vi "Prog_Revision_Date.vi"(5 "Input string":string) -> (0 "Revision time (s)":u32, 2 "svnBaseRevision":u32, 3 "Prog's last revision date":string)   [LabVIEW 2011]
uses:
  <vilib>/Utility/miscctls.llb/LVDateTimeRec.ctl
panel:
  out "source":string
  out "Prog's last revision time":string
  out "RevisionData":string
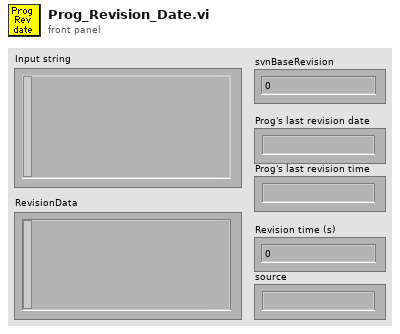
[diagram p1: front panel]
types:
  T1 = typedef "LVDateTimeRec.ctl" = cluster{"fractional second":dbl, "second":i32, "minute":i32, "hour":i32, "day of month":i32, "month":i32, "year":i32, "day of week":i32, "day of year":i32, "DST":i32}
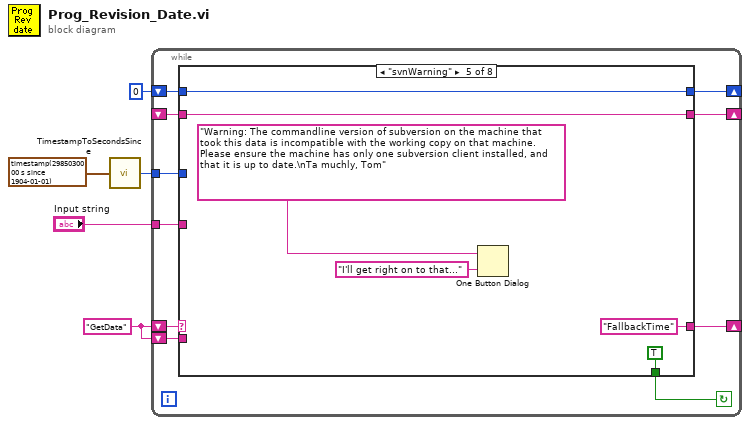
[diagram p0: block diagram]
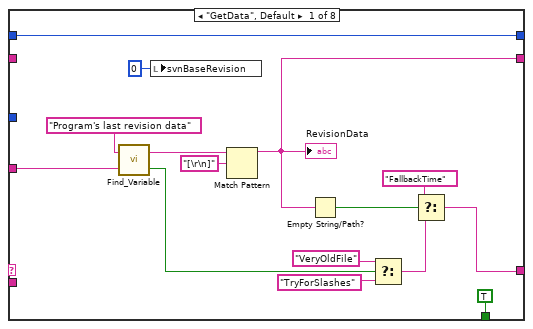
[diagram p2: hidden frame]
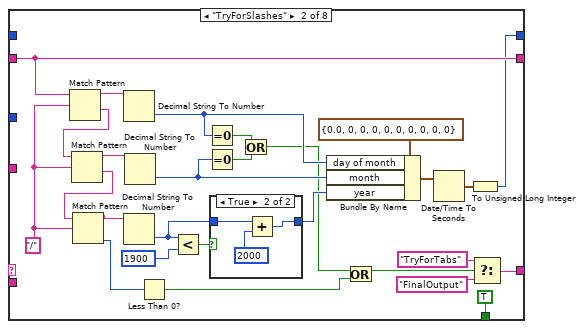
[diagram p3: hidden frame]
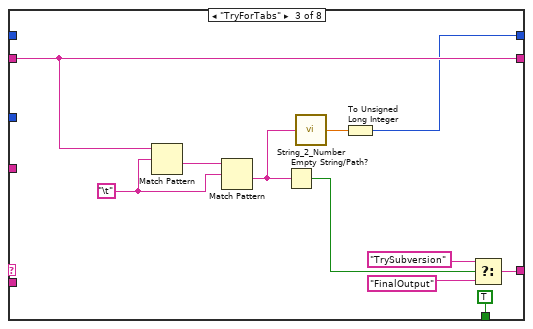
[diagram p5: hidden frame]
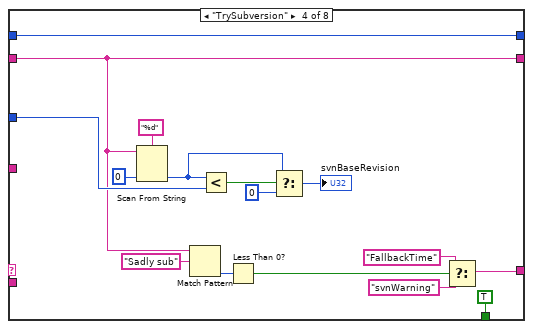
[diagram p6: hidden frame]
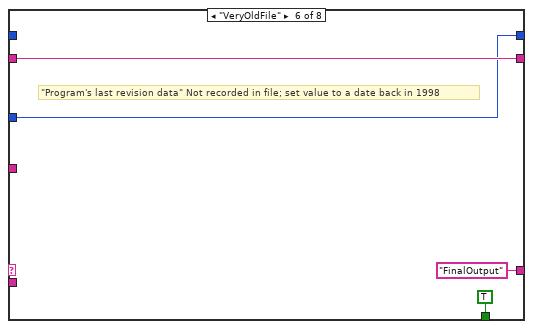
[diagram p7: hidden frame]
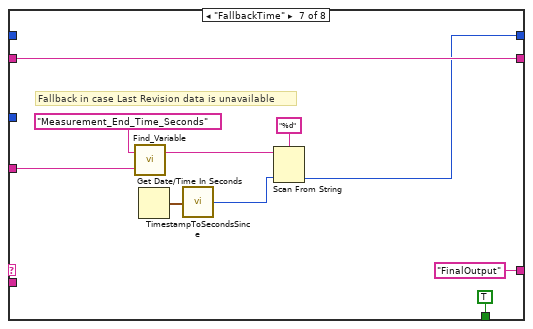
[diagram p8: hidden frame]
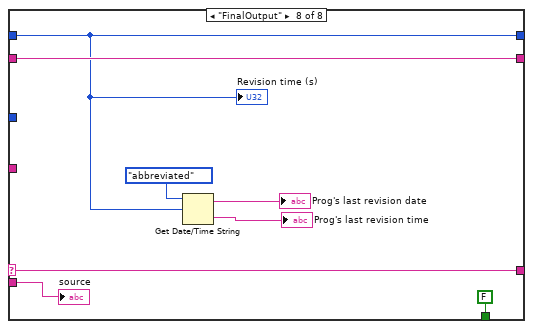
[diagram p9: hidden frame]
diagram:
  w1 = "GetData"
  n1 = call "TimestampToSecondsSince.vi"("Time Stamp Control"=timestamp(2985030000 s since 1904-01-01)) -> ("unsigned 32bit integer"=w2:u32)
  n2 = while {
    tunnel: "Input string" -> [w15]
    shift-right: [w13] -> _
    shift-left: w1 -> [w14]
    shift-right: [w12] -> _
    shift-left: u32 0 -> [w11]
    shift-right: [w9] -> _
    shift-left: _ -> [w8]
    tunnel: w2 -> [w7]
    shift-left: w1 -> [w6]
    stop <- w10 continue-if-true
    n3 = case shown="\"svnWarning\"" w14 {
      selector: w14 -> [_ _ _ _ _ _ _ w110]
      tunnel: w15 -> [w27 _ _ _ _ _ w104 _]
      tunnel: [w18 w41 w69 w76 "FallbackTime" ("t") "FinalOutput" "FinalOutput" w110] -> w13
      tunnel: [w24 w43 w63 w88 w94 w95 w101 w112] -> w12
      tunnel: w11 -> [w24 _ _ w88 w94 _ _ w112]
      tunnel: [TRUE TRUE TRUE TRUE TRUE TRUE TRUE FALSE] -> w10
      tunnel: [w21 w44 w70 w79 w93 w96 w108 w116] -> w9
      tunnel: w8 -> [_ w44 w70 w79 w93 w96 w108 w116]
      tunnel: w7 -> [_ _ _ w85 _ w95 _ _]
      tunnel: w6 -> [_ _ _ _ _ _ _ w109]
      frame "GetData", Default {
        n4 = call "Find_Variable.vi"("Input string"=w27, "Variable name"="Program's last revision data") -> ("No Match?"=w26:bool, "After  Matched string"=w29:string)
        n5 = local write "svnBaseRevision"(0 ("svnBaseRevision")) -> ()
        n6 = Match Pattern(string=w29, regular expression="[\r\n]") -> (before substring=w21:string)  [unwired: 4 out]
        "RevisionData" <- w21
        n7 = Empty String/Path?(string/path=w21) -> (empty?=w19:bool)
        n8 = Select(t="VeryOldFile", s=w26, f="TryForSlashes") -> (s? t:f=w20:string)
        n9 = Select(t="FallbackTime", s=w19, f=w20) -> (s? t:f=w18:string)
      }
      frame "TryForSlashes" {
        w45 = "/" ("search char (-)")
        n10 = Match Pattern(string=w44, regular expression=w45) -> (before substring=w46:string, after substring=w47:string)  [unwired: 3 out]
        n11 = Match Pattern(string=w47, regular expression=w45) -> (before substring=w48:string, after substring=w50:string)  [unwired: 3 out]
        n12 = Match Pattern(string=w50, regular expression=w45) -> (before substring=w49:string, offset past match=w39:i32)  [unwired: 3 out]
        n13 = Decimal String To Number(string=w46) -> (number=w37:i32)  [unwired: 3 out]
        n14 = Decimal String To Number(string=w49) -> (number=w54:i32)  [unwired: 3 out]
        n15 = Decimal String To Number(string=w48) -> (number=w36:i32)  [unwired: 3 out]
        n16 = Less Than 0?(x=w39) -> (x < 0?=w32:bool)
        n17 = Less?(x=w54, y=1900) -> (x < y?=w53:bool)
        n18 = Equal To 0?(x=w37) -> (x = 0?=w35:bool)
        n19 = Equal To 0?(x=w36) -> (x = 0?=w34:bool)
        n20 = case shown="True" w53 {
          tunnel: w54 -> [w58 w60]
          tunnel: [w58 w59] -> w55
          frame False {
          }
          frame True {
            n21 = Add(x=w60, y=2000) -> (x+y=w59:i32)
          }
        }
        n22 = Or(x=w35, y=w34) -> (x .or. y?=w31:bool)
        n23 = Bundle By Name(cluster=T1 {"fractional second"=0.0, "second"=0, "minute"=0, "hour"=0, "day of month"=0, "month"=0, "year"=0, "day of week"=0, "day of year"=0, "DST"=0} ("date time rec"), "day of month"=w37, "month"=w36, "year"=w55) -> (w57:T1)
        n24 = Or(x=w31, y=w32) -> (x .or. y?=w33:bool)
        n25 = Date/Time To Seconds(2:w57) -> (0:w51:timestamp)  [unwired: 1 in]
        n26 = To Unsigned Long Integer(number=w51) -> (unsigned 32bit integer=w43:u32)
        n27 = Select(t="TryForTabs", s=w33, f="FinalOutput") -> (s? t:f=w41:string)
      }
      frame "TryForTabs" {
        w72 = "\t"
        n28 = Match Pattern(string=w70, regular expression=w72) -> (after substring=w71:string)  [unwired: 4 out]
        n29 = Match Pattern(string=w71, regular expression=w72) -> (after substring=w64:string)  [unwired: 4 out]
        n30 = Empty String/Path?(string/path=w64) -> (empty?=w68:bool)
        n31 = call "String_2_Number.vi"("Value"=w64) -> ("Numeric"=w65:dbl)
        n32 = To Unsigned Long Integer(number=w65) -> (unsigned 32bit integer=w63:u32)
        n33 = Select(t="TrySubversion", s=w68, f="FinalOutput") -> (s? t:f=w69:string)
      }
      frame "TrySubversion" {
        n34 = Scan From String(format string="%d", input string=w79, default 1=u32 0 ("unsigned 32bit integer")) -> (output 1=w83:u32)  [unwired: 2 in, 3 out]
        n35 = Match Pattern(string=w79, regular expression="Sadly sub") -> (offset past match=w77:i32)  [unwired: 1 in, 3 out]
        n36 = Less?(x=w83, y=w85) -> (x < y?=w84:bool)
        n37 = Less Than 0?(x=w77) -> (x < 0?=w74:bool)
        n38 = Select(t=w83, s=w84, f=u32 0) -> (s? t:f=→"svnBaseRevision":u32)
        n39 = Select(t="FallbackTime", s=w74, f="svnWarning" ("t")) -> (s? t:f=w76:string)
      }
      frame "svnWarning" {
        n40 = One Button Dialog(message="Warning: The commandline version of subversion on the machine that took this data is incompatible with the working copy on that machine. Please ensure the machine has only one subversion client installed, and that it is up to date.\nTa muchly, Tom", button name ("OK")="I'll get right on to that...") -> ()  [unwired: 1 out]
      }
      frame "VeryOldFile" {
        # "\"Program's last revision data\" Not recorded in file; set value to a date back in 1998"
      }
      frame "FallbackTime" {
        # "Fallback in case Last Revision data is unavailable"
        n41 = call "Find_Variable.vi"("Input string"=w104, "Variable name"="Measurement_End_Time_Seconds") -> ("After  Matched string"=w105:string)  [unwired: 1 out]
        n42 = Get Date/Time In Seconds() -> (seconds since 1Jan1904=w100:timestamp)
        n43 = call "TimestampToSecondsSince.vi"("Time Stamp Control"=w100) -> ("unsigned 32bit integer"=w99:u32)
        n44 = Scan From String(format string="%d", input string=w105, default 1=w99) -> (output 1=w101:u32)  [unwired: 2 in, 3 out]
      }
      frame "FinalOutput" {
        n45 = Get Date/Time String(date format (0)=enum16{"short", "long", "abbreviated"}."abbreviated", seconds (now)=w112) -> (date string=→"Prog's last revision date":string, time string=→"Prog's last revision time":string)  [unwired: 1 out]
        "Revision time (s)" <- w112
        "source" <- w109
      }
    }
  }
